vi "initialize_magnetometer.vi"(0 "magnetometer in":refnum<class "magnetometer.lvclass">, 1 "sampling info":cluster{"Fs":dbl, "#s":dbl}, 5 "mag inputs":T1, 11 "error in (no error)":errorcluster) -> (4 "magnetometer out":refnum<class "magnetometer.lvclass">, 15 "error out":errorcluster)   [LabVIEW 2015, in "magnetometer.lvclass"]
uses:
  magnetometer.lvclass
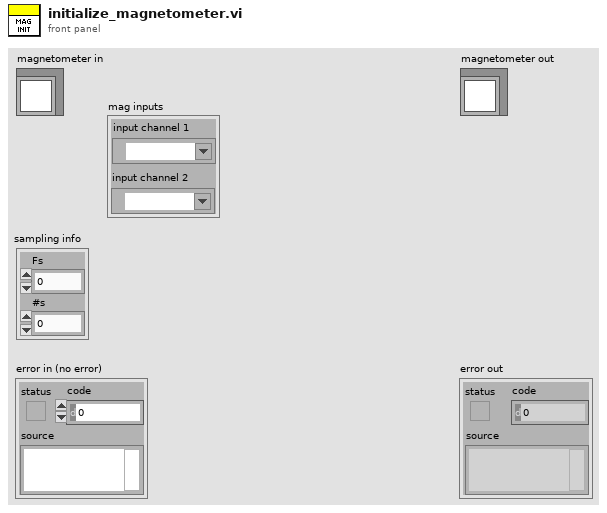
[diagram p1: front panel]
types:
  T1 = cluster{"input channel 1":tag, "input channel 2":tag}
  T2 = cluster{"task out":refnum<k21>, "task out":refnum<k21>}
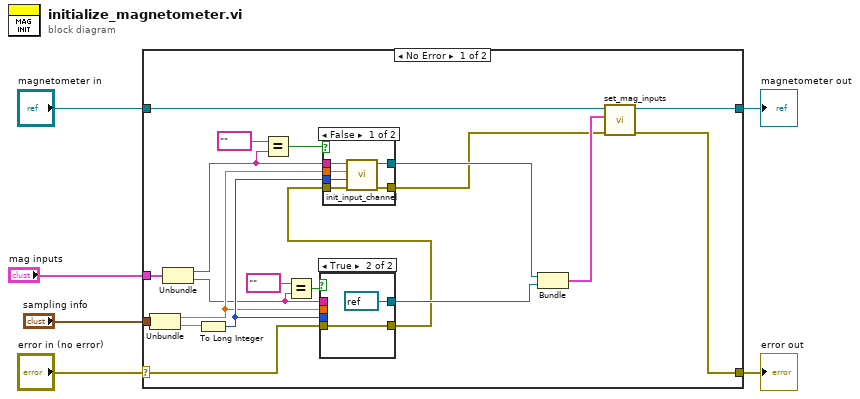
[diagram p0: block diagram]
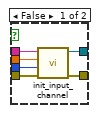
[diagram p2: hidden frame]
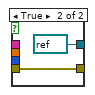
[diagram p3: hidden frame]
diagram:
  n1 = case shown="No Error" "error in (no error)" {
    selector: "error in (no error)" -> [w16 w44]
    tunnel: [w13 w44] -> w5
    tunnel: [w17 w43] -> w3
    tunnel: "magnetometer in" -> [w18 w43]
    tunnel: "sampling info" -> [w25 _]
    tunnel: "mag inputs" -> [w22 _]
    frame No Error {
      n2 = Unbundle(w25) -> ("Fs"=w23:dbl, "#s"=w26:dbl)
      n3 = Unbundle(w22) -> ("input channel 1"=w12:tag, "input channel 2"=w7:tag)
      n4 = To Long Integer(number=w26) -> (32bit integer=w24:i32)
      n5 = Equal?(x=tag "", y=w12) -> (x = y?=w11:bool)
      n6 = Equal?(x=tag "", y=w7) -> (x = y?=w8:bool)
      n7 = case shown="True" w8 {
        tunnel: w24 -> [w32 _]
        tunnel: w23 -> [w31 _]
        tunnel: w7 -> [w30 _]
        tunnel: [w29 refnum<k21> refnum ("task out")] -> w20
        tunnel: w16 -> [w28 w34]
        tunnel: [w27 w34] -> w15
        frame False {
          n8 = call "init_input_channel.vi"("error in (no error)"=w28, "samples per channel"=w32, "rate"=w31, "input channel"=w30) -> ("error out"=w27:errorcluster, "task out"=w29:refnum<k21>)  [unwired: 6 in]
        }
        frame True {
        }
      }
      n9 = case shown="False" w11 {
        tunnel: w24 -> [w40 _]
        tunnel: w23 -> [w39 _]
        tunnel: w12 -> [w38 _]
        tunnel: [w37 refnum<k21> refnum ("task out")] -> w21
        tunnel: w15 -> [w36 w42]
        tunnel: [w35 w42] -> w14
        frame False {
          n10 = call "init_input_channel.vi"("error in (no error)"=w36, "samples per channel"=w40, "rate"=w39, "input channel"=w38) -> ("error out"=w35:errorcluster, "task out"=w37:refnum<k21>)  [unwired: 6 in]
        }
        frame True {
        }
      }
      n11 = Bundle("task out"=w21, "task out"=w20) -> (w19:T2)  [unwired: 1 in]
      n12 = call-dynamic "set_mag_inputs.vi"("error in (no error)"=w14, "mag inputs"=w19, "magnetometer in"=w18) -> ("error out"=w13:errorcluster, "magnetometer out"=w17:refnum<class "magnetometer.lvclass">)  [unwired: 7 in]
    }
    frame Error {
    }
  }
  "error out" <- w5
  "magnetometer out" <- w3
